vi "Find String Dialog.vi"(8 "error in (no error)":errorcluster) -> (0 "error out":errorcluster, 1 "Cancelled":bool caption="OK", 3 "String to search (out)":string caption="String to search for:")   [LabVIEW 2021, in "Strings.lvlib"]
doc: "Displays a standard dialog box that prompts users to enter information, such as a user name and password.\n--------------------\n\nThis Express VI is configured as follows:\n\nMessage to Display to the User:\nThe inputs are: \nText Entry Box: String to search for:"
uses:
  Strings/Strings.lvlib
panel:
  in  "String to search:":string caption="String to search for:"
  in  "Cancel":bool
  in  "OK":bool caption="OK2"
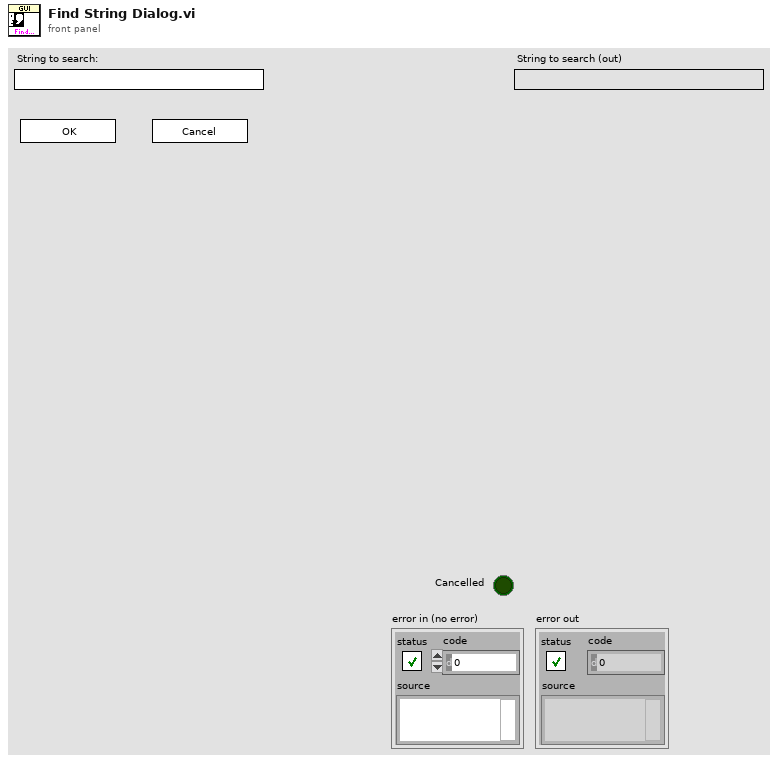
[diagram p1: front panel]
types:
  T1 = enum32{"Invalid", "Standard", "Closed", "Hidden", "Minimized", "Maximized"}
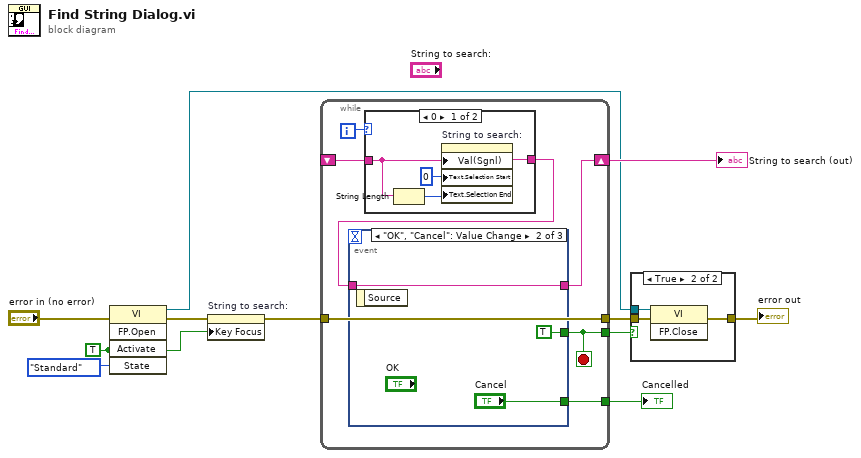
[diagram p0: block diagram]
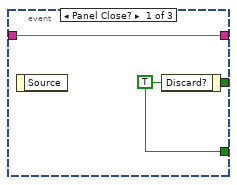
[diagram p3: hidden frame]
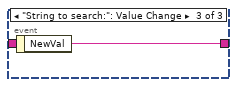
[diagram p4: hidden frame]
diagram:
  w4 = TRUE ("Activate?")
  n1 = invoke class="VI" method="FP.Open"(error in="error in (no error)", "Activate"=w4, "State"=T1."Standard") -> (reference out=w3:refnum<vi>, error out=w11:errorcluster)  [unwired: 2 in, 3 out]
  n2 = property on="String to search:" class="Str"(error in=w11, "Key Focus"=w4) -> (error out=w5:errorcluster)  [unwired: 1 in, 1 out]
  n3 = while {
    tunnel: [w17] -> w9
    tunnel: [w18] -> w6
    tunnel: w5 -> [w16]
    tunnel: [w16] -> w1
    shift-right: [w13] -> w10
    shift-left: _ -> [w14]
    i -> [w15]
    stop <- w17 stop-if-true
    n4 = case shown="0" w15 {
      tunnel: w14 -> [w20 w22]
      tunnel: [w20 w22] -> w12
      frame 0 {
        n5 = String Length(string=w20) -> (length=w19:i32)
        n6 = property on="String to search:" class="Str"("Val(Sgnl)"=w20, "Text.Selection Start"=u32 0 ("Text.Selection:Start"), "Text.Selection End"=w19) -> ()  [unwired: 2 in, 2 out]
      }
      frame 1, Default {
      }
    }
    n7 = event shown="[1] \"OK\", \"Cancel\": Value Change" {
      selector: _ -> [_ _ _]
      dyn-events: _ -> [_ _ _]
      timeout: _ -> [_ _ _]
      tunnel: [w24 TRUE ("Discard?") _] -> w17
      tunnel: [w24 "Cancel" _] -> w18
      tunnel: [w23 w25 w28] -> w13
      tunnel: w12 -> [w23 w25 _]
      event Panel Close? {
        w24 = TRUE ("Discard?")
        n8 = event-data() -> ()  [unwired: 1 in, 1 out]
        n9 = event-data("Discard?"=w24) -> ()  [unwired: 1 in, 1 out]
      }
      event "OK", "Cancel": Value Change {
        n10 = event-data() -> ()  [unwired: 1 in, 1 out]
      }
      event "String to search:": Value Change {
        n11 = event-data() -> ("NewVal"=w28:string)  [unwired: 1 in]
      }
    }
  }
  "Cancelled" <- w6
  "String to search (out)" <- w10
  n12 = case shown="True" w9 {
    tunnel: w3 -> [_ w32]
    tunnel: [w29 w31] -> w2
    tunnel: w1 -> [w29 w30]
    frame False {
    }
    frame True {
      n13 = invoke class="VI" method="FP.Close"(reference=w32, error in=w30) -> (error out=w31:errorcluster)  [unwired: 1 in, 2 out]
    }
  }
  "error out" <- w2
